vi "PWA_Setup_Panel.vi"(0 "Show Panel?":bool, 1 "Check Calib file?":bool, 2 "OK":T1, 3 "Incoming Setup String":string) -> (7 "Outgoing Setup String":string)   [LabVIEW 2022 SP3]
uses:
  Controls/ok_button.ctl
  File/Setup_Filetype.ctl
  Controls/Post_Process.ctl
  Controls/App_Global.ctl
  Controls/Inst_type.ctl
  Globals/Meas_global.vi
  PWAtasksGLOBAL.vi
panel:
  in  "Probe Rotated Thro' 180":bool
  in  "Software + buffering delay per pulse (s)":dbl=9.7e-06
  in  "Symbol":string
  in  "Pulse length \nx2 micro sec":i16=1 min=1 max=12
  in  "Clock Rate":bool
  in  "Gain":i16=1 min=1 max=12
  in  "Wire Current mA":i16(knob)=1 min=1 max=3 step=1 scale=1.0..3.0
  in  "Trigger -ve":dbl(knob)=1.0 min=0.0 max=5.0 scale=0.0..5.0 scale format="%#.2f"
  in  "Trigger +ve":dbl(knob)=1.0 min=0.0 max=5.0 scale=0.0..5.0 scale format="%#.2f"
  out "Calib Path from file":path
  in  "Use Latest":bool=TRUE
  in  "PWA Calib. File Path":path=path "/G5_1_HD/Users/paulhayden/Desktop/Labview test/PWA_Calib.xls"
  in  "Minimum TOF (mu.s)":i16=225
  in  "PWA Freq. (Hz)":dbl=30.0 min=0.0 max=50.0
  # "PELA Flow Instruments Ltd."
  # "TRIGGER LEVELS\n(volts)"
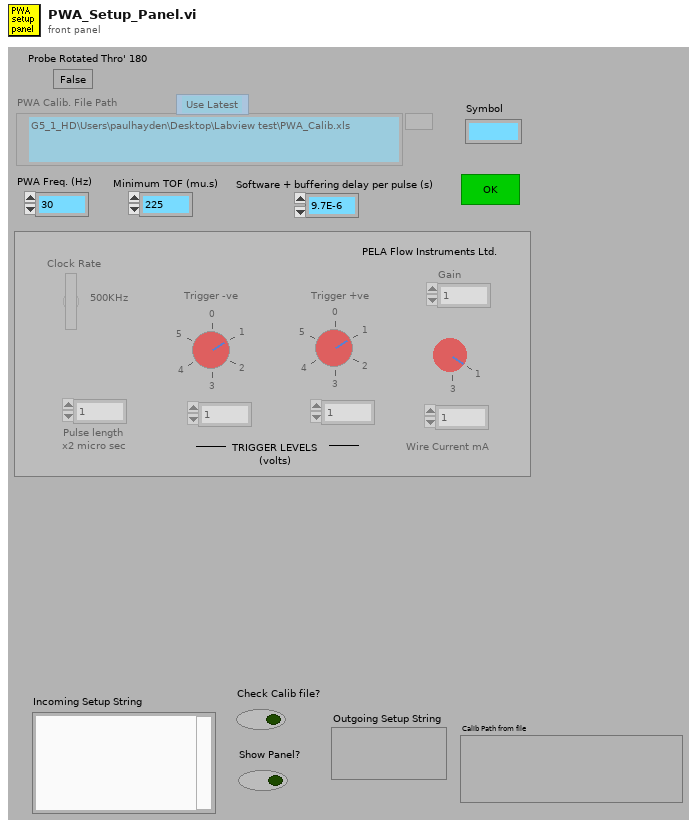
[diagram p1: front panel]
types:
  T1 = typedef "ok_button.ctl" = bool
  T2 = typedef "Setup_Filetype.ctl" = enum16{"Measurement Setups", "Calibration Setups", "General", "Results File Plotter Setups", "Speed Calib Tweaks"}
  T3 = typedef "Post_Process.ctl" = enum16{"Take New Data", "Post Process Raw Data File"}
  T4 = typedef "App_Global.ctl" = enum16{"Read Global", "Write to Global", "Initialise Array"}
  T5 = typedef "Inst_type.ctl" = enum16{"Raw voltage", "Raw with zero offsetting", "Propeller anemometer", "Pressure Transducer", "Pitot-static tube", "Hot wire", "Cross wire 1", "Cross wire 2", "Generic Linear", "Generic Polynomial", "Generic BackPoly", "Fast FID", "Thermocouple", "Cold wire", "Pulsed Wire", "LDA Vel", "LDA Tran time", "LDA Arr time", "Microphone"}
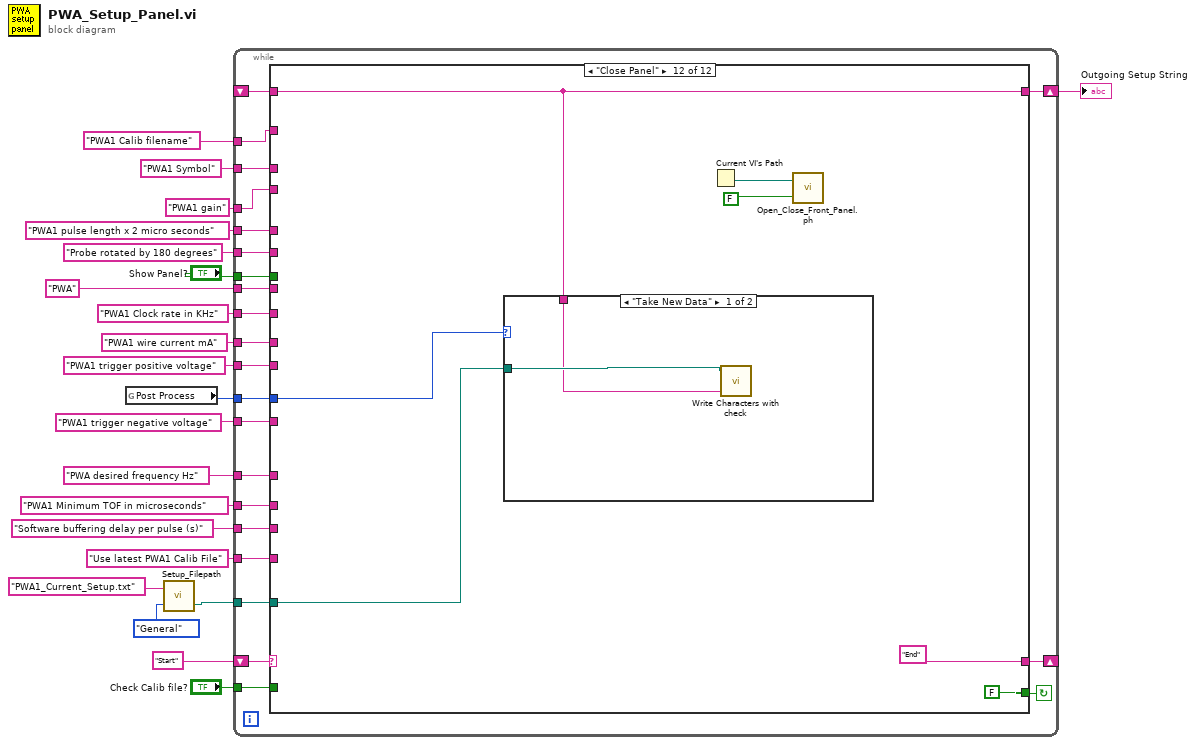
[diagram p0: block diagram]
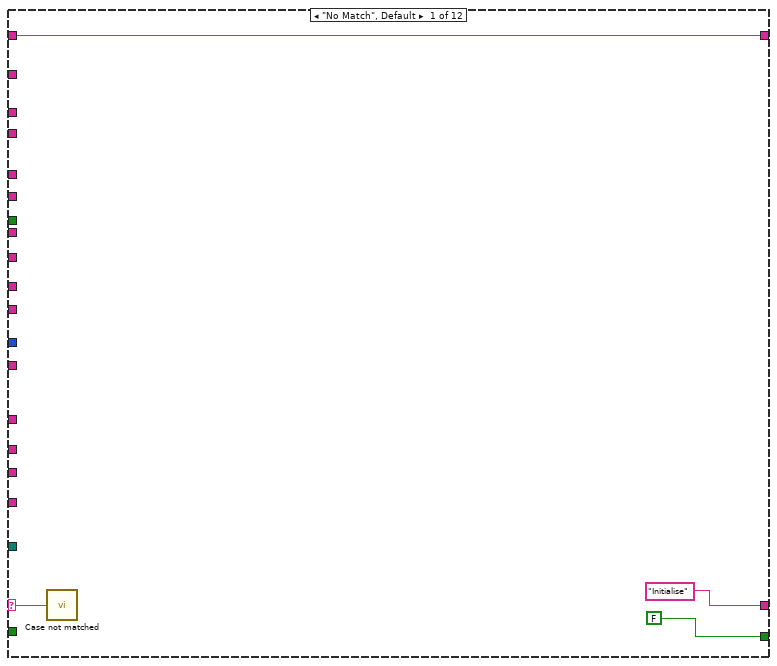
[diagram p2: hidden frame]
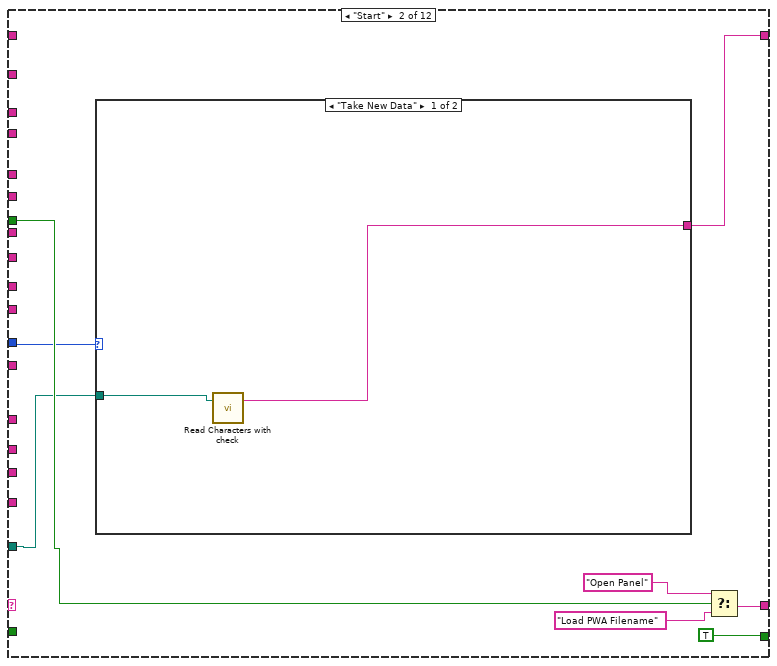
[diagram p3: hidden frame]
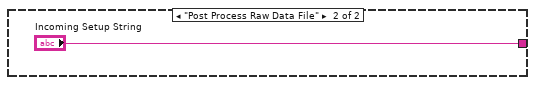
[diagram p4: hidden frame]
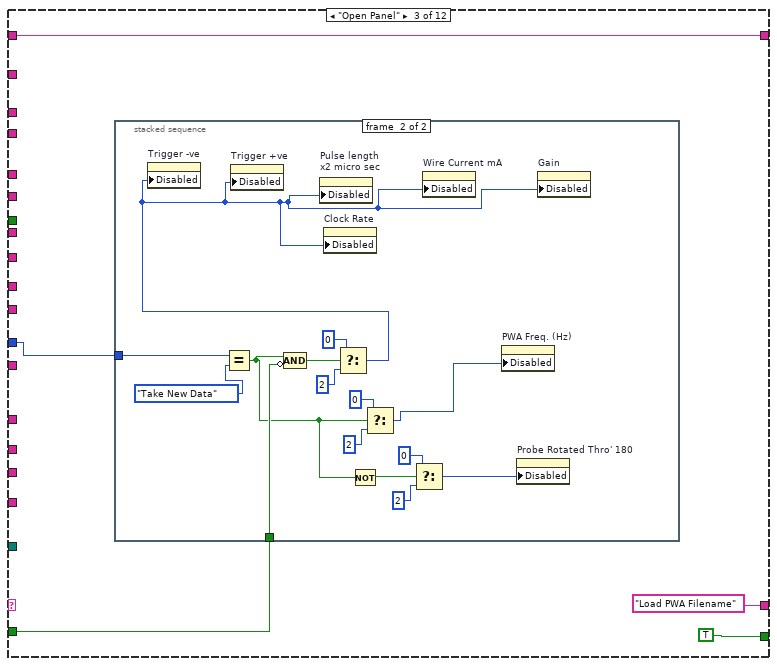
[diagram p5: hidden frame]
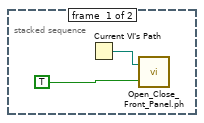
[diagram p6: hidden frame]
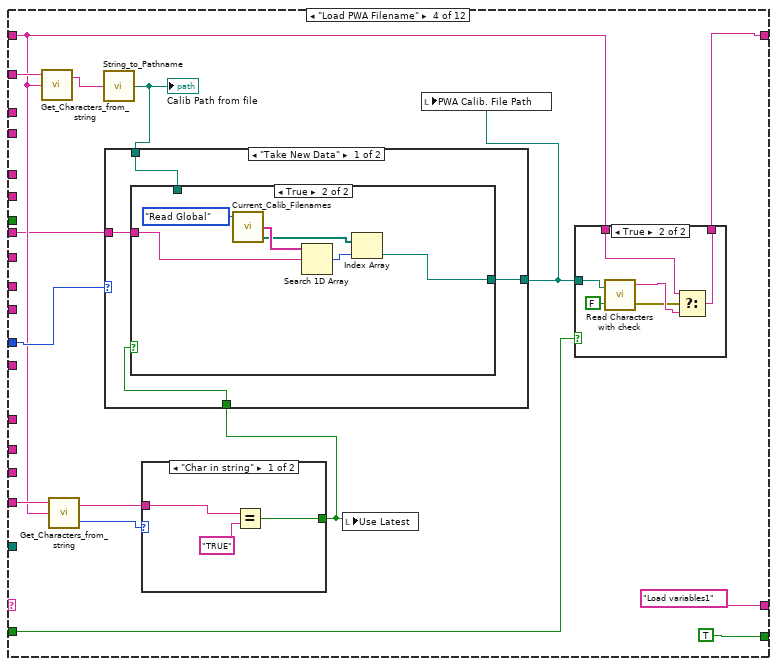
[diagram p7: hidden frame]
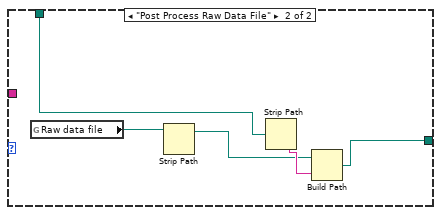
[diagram p10: hidden frame]
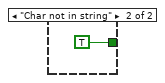
[diagram p11: hidden frame]
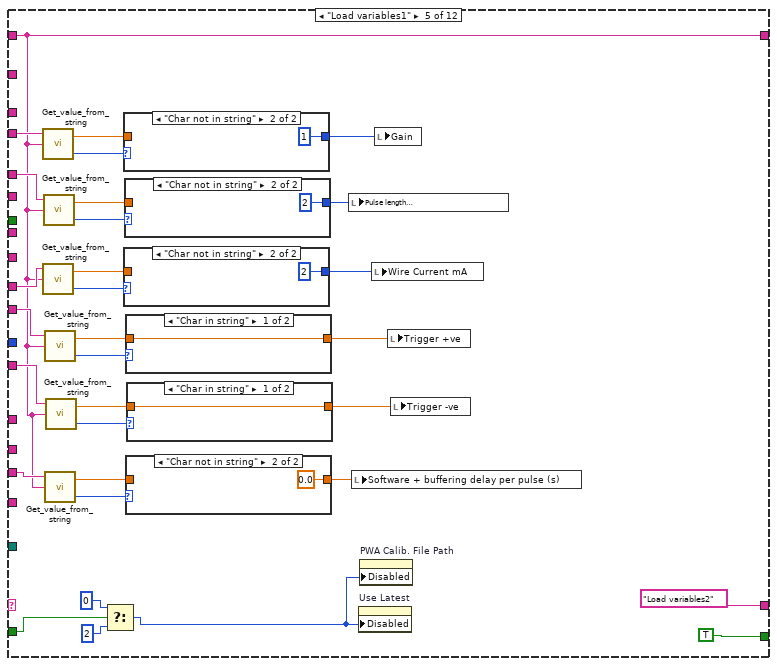
[diagram p12: hidden frame]
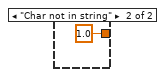
[diagram p14: hidden frame]
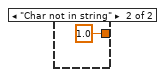
[diagram p15: hidden frame]
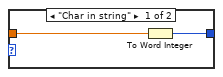
[diagram p16: hidden frame]
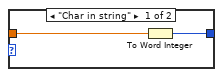
[diagram p17: hidden frame]
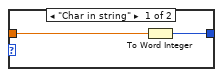
[diagram p18: hidden frame]
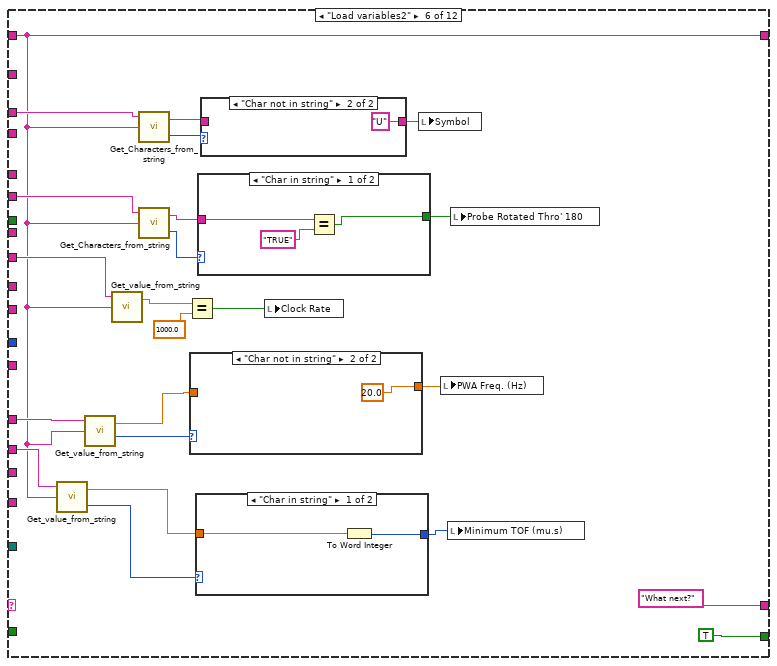
[diagram p19: hidden frame]
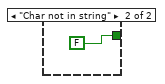
[diagram p20: hidden frame]
diagram:
  n1 = global read "Meas_global.vi" "Post Process"() -> (w20:T3)
  n2 = call "Setup_Filepath.vi"("Setup File Type"=Setup_Filetype."General", "Filename in"="PWA1_Current_Setup.txt" ("name or relative path")) -> ("Filename Out"=w2:path)  [unwired: 1 out]
  n3 = while {
    shift-left: "Start" -> [w43]
    shift-right: [w44] -> _
    tunnel: "Show Panel?" -> [w42]
    tunnel: w20 -> [w41]
    tunnel: "PWA1 Calib filename" -> [w39]
    tunnel: "Use latest PWA1 Calib File" -> [w40]
    tunnel: "PWA1 Minimum TOF in microseconds" -> [w38]
    tunnel: "PWA desired frequency Hz" -> [w37]
    tunnel: "Check Calib file?" -> [w36]
    tunnel: "PWA1 gain" -> [w35]
    tunnel: "PWA1 pulse length x 2 micro seconds" -> [w34]
    tunnel: "PWA1 wire current mA" -> [w33]
    tunnel: "PWA1 trigger positive voltage" -> [w32]
    tunnel: "PWA1 trigger negative voltage" -> [w31]
    tunnel: "PWA1 Clock rate in KHz" -> [w30]
    shift-right: [w29] -> w7
    shift-left: _ -> [w28]
    tunnel: "PWA1 Symbol" -> [w27]
    tunnel: w2 -> [w26]
    tunnel: "Software buffering delay per pulse (s)" -> [w25]
    tunnel: "Probe rotated by 180 degrees" -> [w24]
    tunnel: "PWA" ("element") -> [w23]
    stop <- w45 continue-if-true
    n4 = case shown="\"Close Panel\"" w43 {
      selector: w43 -> [w46 _ _ _ _ _ _ _ _ _ _ _]
      tunnel: [FALSE TRUE TRUE TRUE TRUE TRUE TRUE TRUE ("Show Panel?") TRUE ("Show Panel?") TRUE ("Show Panel?") w334 FALSE ("Show Panel?")] -> w45
      tunnel: ["Initialise" w50 "Load PWA Filename" "Load variables1" "Load variables2" "What next?" w212 "Save PWA values" "2nd Save PWA values" "PWA Setup Summary" "Close Panel" "End"] -> w44
      tunnel: w42 -> [_ w56 _ _ _ _ _ _ _ _ w334 _]
      tunnel: w41 -> [_ w53 w63 w89 _ _ w214 _ _ _ _ w336]
      tunnel: w40 -> [_ _ _ w91 _ _ _ _ w272 _ _ _]
      tunnel: w39 -> [_ _ _ w94 _ _ _ _ w282 _ _ _]
      tunnel: w38 -> [_ _ _ _ _ w191 _ _ w280 _ _ _]
      tunnel: w37 -> [_ _ _ _ _ w190 _ _ w281 _ _ _]
      tunnel: w36 -> [_ _ w61 w86 w153 _ w210 _ _ _ _ _]
      tunnel: w35 -> [_ _ _ _ w146 _ _ _ _ w319 _ _]
      tunnel: w34 -> [_ _ _ _ w142 _ _ _ _ w303 _ _]
      tunnel: w33 -> [_ _ _ _ w130 _ _ _ _ w308 _ _]
      tunnel: w32 -> [_ _ _ _ w135 _ _ _ _ w305 _ _]
      tunnel: w31 -> [_ _ _ _ w131 _ _ _ _ w304 _ _]
      tunnel: w30 -> [_ _ _ _ _ w183 _ _ _ w314 _ _]
      tunnel: [w47 w52 w62 w84 w126 w174 w209 w244 w268 w294 w324 w340] -> w29
      tunnel: w28 -> [w47 _ w62 w85 w126 w174 w209 w244 _ w295 w324 w340]
      tunnel: w27 -> [_ _ _ _ _ w179 _ _ w266 _ _ _]
      tunnel: w26 -> [_ w51 _ _ _ _ _ _ _ _ _ w339]
      tunnel: w25 -> [_ _ _ _ w127 _ _ _ _ w292 _ _]
      tunnel: w24 -> [_ _ _ _ _ w175 _ _ w259 _ _ _]
      tunnel: w23 -> [_ _ _ w83 _ _ w205 w239 _ _ _ _]
      frame "No Match", Default {
        n5 = call "Case not matched.vi"("Case Name not Matched"=w46) -> ()
      }
      frame "Start" {
        n6 = case shown="\"Take New Data\"" w53 {
          tunnel: [w58 "Incoming Setup String"] -> w52
          tunnel: w51 -> [w59 _]
          frame "Take New Data" {
            n7 = call "Read Characters with check.vi"("file (use dialog)"=w59) -> ("Read String"=w58:string)  [unwired: 1 in, 1 out]
          }
          frame "Post Process Raw Data File" {
          }
        }
        n8 = Select(t="Open Panel", s=w56, f="Load PWA Filename") -> (s? t:f=w50:string)
      }
      frame "Open Panel" {
        n9 = stacked-sequence {
          tunnel: w63 -> [_ w82]
          tunnel: w61 -> [_ w77]
          frame #0 {
            n10 = Current VI's Path() -> (path=w67:path)
            n11 = call "Open_Close_Front_Panel.ph.vi"("openWindow (T)"=TRUE ("Front Panel Window:Open"), "VI path"=w67) -> ()  [unwired: 1 in, 1 out]
          }
          frame #1 {
            n12 = Equal?(x=w82, y=Post_Process."Take New Data" ("Post Process")) -> (x = y?=w70:bool)
            n13 = Compound Arithmetic op=AND(w70, invert w77) -> (w76:bool)
            n14 = Select(t=u8 0 ("Disabled"), s=w76, f=u8 2) -> (s? t:f=w78:u8)
            n15 = property on="Trigger -ve" class="Knob (strict)"("Disabled"=w78) -> ()  [unwired: 2 in, 2 out]
            n16 = property on="Trigger +ve" class="Knob (strict)"("Disabled"=w78) -> ()  [unwired: 2 in, 2 out]
            n17 = property on="Pulse length \nx2 micro sec" class="DigNum (strict)"("Disabled"=w78) -> ()  [unwired: 2 in, 2 out]
            n18 = property on="Clock Rate" class="Bool (strict)"("Disabled"=w78) -> ()  [unwired: 2 in, 2 out]
            n19 = Not(x=w70) -> (.not. x?=w69:bool)
            n20 = Select(t=u8 0 ("Disabled"), s=w70, f=u8 2) -> (s? t:f=w73:u8)
            n21 = Select(t=u8 0 ("Disabled"), s=w69, f=u8 2) -> (s? t:f=w68:u8)
            n22 = property on="Wire Current mA" class="Knob (strict)"("Disabled"=w78) -> ()  [unwired: 2 in, 2 out]
            n23 = property on="PWA Freq. (Hz)" class="DigNum (strict)"("Disabled"=w73) -> ()  [unwired: 2 in, 2 out]
            n24 = property on="Probe Rotated Thro' 180" class="Bool (strict)"("Disabled"=w68) -> ()  [unwired: 2 in, 2 out]
            n25 = property on="Gain" class="DigNum (strict)"("Disabled"=w78) -> ()  [unwired: 2 in, 2 out]
          }
        }
      }
      frame "Load PWA Filename" {
        n26 = call "Get_Characters_from_string.vi"("Input string"=w85, "Variable name"=w94) -> ("Value"=w95:string)  [unwired: 1 in, 1 out]
        n27 = call "Get_Characters_from_string.vi"("Input string"=w85, "Variable name"=w91) -> ("Status"=w92:enum16{"Char in string", "Char not in string"}, "Value"=w93:string)  [unwired: 1 in]
        n28 = call "String_to_Pathname.vi"("Input String"=w95) -> ("path"=w90:path)
        "Calib Path from file" <- w90
        n29 = case shown="\"Char in string\"" w92 {
          tunnel: w93 -> [w123 _]
          tunnel: [w121 TRUE] -> w88
          frame "Char in string" {
            n30 = Equal?(x=w123, y="TRUE") -> (x = y?=w121:bool)
          }
          frame "Char not in string" {
          }
        }
        n31 = case shown="\"Take New Data\"" w89 {
          tunnel: [w107 w116] -> w87
          tunnel: w90 -> [w106 w119]
          tunnel: w88 -> [w108 _]
          tunnel: w83 -> [w105 _]
          frame "Take New Data" {
            n32 = case shown="True" w108 {
              tunnel: [w109 w111] -> w107
              tunnel: w106 -> [w109 _]
              tunnel: w105 -> [_ w110]
              frame False {
              }
              frame True {
                n33 = call "Current_Calib_Filenames.vi"("Mode"=App_Global."Read Global") -> ("Calib Filename Out"=w113:path[], "Channel ID Output"=w114:string[])  [unwired: 2 in, 1 out]
                n34 = Search 1D Array(1D array=w114, element=w110) -> (index of element=w112:i32)  [unwired: 1 out]
                n35 = Index Array(array=w113, index=w112) -> (element=w111:path)
              }
            }
          }
          frame "Post Process Raw Data File" {
            n36 = global read "Meas_global.vi" "Raw data file"() -> (w120:path)
            n37 = Strip Path(path=w120) -> (stripped path=w117:path)  [unwired: 1 out]
            n38 = Strip Path(path=w119) -> (name=w118:string)  [unwired: 1 out]
            n39 = Build Path(base path=w117, name or relative path=w118) -> (appended path=w116:path)
          }
        }
        n40 = local write "Use Latest"(w88) -> ()
        n41 = local write "PWA Calib. File Path"(w87) -> ()
        n42 = case shown="True" w86 {
          tunnel: w87 -> [_ w100]
          tunnel: w85 -> [w98 w104]
          tunnel: [w98 w103] -> w84
          frame False {
          }
          frame True {
            n43 = call "Read Characters with check.vi"("Call EnFlo Error Handler?"=FALSE, "file (use dialog)"=w100) -> ("error out"=w101:errorcluster, "Read String"=w102:string)
            n44 = Select(t=w104, s=w101, f=w102) -> (s? t:f=w103:string)
          }
        }
      }
      frame "Load variables1" {
        n45 = call "Get_value_from_string.vi"("Input string"=w126, "Variable name"=w146) -> ("Status"=w148:enum16{"Char in string", "Char not in string"}, "Value"=w149:dbl)  [unwired: 1 in]
        n46 = call "Get_value_from_string.vi"("Input string"=w126, "Variable name"=w130) -> ("Status"=w140:enum16{"Char in string", "Char not in string"}, "Value"=w141:dbl)  [unwired: 1 in]
        n47 = call "Get_value_from_string.vi"("Input string"=w126, "Variable name"=w142) -> ("Status"=w144:enum16{"Char in string", "Char not in string"}, "Value"=w143:dbl)  [unwired: 1 in]
        n48 = call "Get_value_from_string.vi"("Input string"=w126, "Variable name"=w135) -> ("Status"=w137:enum16{"Char in string", "Char not in string"}, "Value"=w136:dbl)  [unwired: 1 in]
        n49 = call "Get_value_from_string.vi"("Input string"=w126, "Variable name"=w127) -> ("Status"=w128:enum16{"Char in string", "Char not in string"}, "Value"=w125:dbl)  [unwired: 1 in]
        n50 = call "Get_value_from_string.vi"("Input string"=w126, "Variable name"=w131) -> ("Status"=w133:enum16{"Char in string", "Char not in string"}, "Value"=w134:dbl)  [unwired: 1 in]
        n51 = Select(t=u8 0 ("Disabled"), s=w153, f=u8 2 ("Disabled")) -> (s? t:f=w150:u8)
        n52 = case shown="\"Char not in string\"" w148 {
          tunnel: w149 -> [w169 _]
          tunnel: [w168 i16 1 ("PWA No. of Samples")] -> w147
          frame "Char in string" {
            n53 = To Word Integer(number=w169) -> (16bit integer=w168:i16)
          }
          frame "Char not in string" {
          }
        }
        n54 = case shown="\"Char not in string\"" w140 {
          tunnel: w141 -> [w163 _]
          tunnel: [w162 i16 2 ("PWA No. of Samples")] -> w139
          frame "Char in string" {
            n55 = To Word Integer(number=w163) -> (16bit integer=w162:i16)
          }
          frame "Char not in string" {
          }
        }
        n56 = case shown="\"Char not in string\"" w144 {
          tunnel: w143 -> [w166 _]
          tunnel: [w165 i16 2 ("PWA No. of Samples")] -> w145
          frame "Char in string" {
            n57 = To Word Integer(number=w166) -> (16bit integer=w165:i16)
          }
          frame "Char not in string" {
          }
        }
        n58 = case shown="\"Char in string\"" w137 {
          tunnel: w136 -> [w160 _]
          tunnel: [w160 1.0 ("Value")] -> w138
          frame "Char in string" {
          }
          frame "Char not in string" {
          }
        }
        n59 = case shown="\"Char not in string\"" w128 {
          tunnel: w125 -> [w156 _]
          tunnel: [w156 0.0 ("Value")] -> w129
          frame "Char in string" {
          }
          frame "Char not in string" {
          }
        }
        n60 = case shown="\"Char in string\"" w133 {
          tunnel: w134 -> [w158 _]
          tunnel: [w158 1.0 ("Value")] -> w132
          frame "Char in string" {
          }
          frame "Char not in string" {
          }
        }
        n61 = local write "Pulse length \nx2 micro sec"(w145) -> ()
        n62 = local write "Software + buffering delay per pulse (s)"(w129) -> ()
        n63 = property on="Use Latest" class="Bool (strict)"("Disabled"=w150) -> ()  [unwired: 2 in, 2 out]
        n64 = property on="PWA Calib. File Path" class="Path"("Disabled"=w150) -> ()  [unwired: 2 in, 2 out]
        n65 = local write "Wire Current mA"(w139) -> ()
        n66 = local write "Gain"(w147) -> ()
        n67 = local write "Trigger +ve"(w138) -> ()
        n68 = local write "Trigger -ve"(w132) -> ()
      }
      frame "Load variables2" {
        n69 = call "Get_value_from_string.vi"("Input string"=w174, "Variable name"=w191) -> ("Status"=w186:enum16{"Char in string", "Char not in string"}, "Value"=w185:dbl)  [unwired: 1 in]
        n70 = call "Get_value_from_string.vi"("Input string"=w174, "Variable name"=w190) -> ("Status"=w189:enum16{"Char in string", "Char not in string"}, "Value"=w188:dbl)  [unwired: 1 in]
        n71 = call "Get_value_from_string.vi"("Input string"=w174, "Variable name"=w183) -> ("Value"=w182:dbl)  [unwired: 1 in, 1 out]
        n72 = call "Get_Characters_from_string.vi"("Input string"=w174, "Variable name"=w179) -> ("Status"=w178:enum16{"Char in string", "Char not in string"}, "Value"=w177:string)  [unwired: 1 in]
        n73 = call "Get_Characters_from_string.vi"("Input string"=w174, "Variable name"=w175) -> ("Status"=w173:enum16{"Char in string", "Char not in string"}, "Value"=w171:string)  [unwired: 1 in]
        n74 = Equal?(x=w182, y=1000.0) -> (x = y?=w180:bool)
        n75 = case shown="\"Char not in string\"" w189 {
          tunnel: w188 -> [w203 _]
          tunnel: [w203 20.0 ("PWA No. of Samples")] -> w187
          frame "Char in string" {
          }
          frame "Char not in string" {
          }
        }
        n76 = case shown="\"Char in string\"" w186 {
          tunnel: w185 -> [w201 _]
          tunnel: [w200 i16 225 ("Minimum TOF (mu.s)")] -> w184
          frame "Char in string" {
            n77 = To Word Integer(number=w201) -> (16bit integer=w200:i16)
          }
          frame "Char not in string" {
          }
        }
        n78 = case shown="\"Char in string\"" w173 {
          tunnel: [w194 FALSE] -> w172
          tunnel: w171 -> [w196 _]
          frame "Char in string" {
            n79 = Equal?(x=w196, y="TRUE") -> (x = y?=w194:bool)
          }
          frame "Char not in string" {
          }
        }
        n80 = case shown="\"Char not in string\"" w178 {
          tunnel: w177 -> [w198 _]
          tunnel: [w198 "U" ("Value")] -> w176
          frame "Char in string" {
          }
          frame "Char not in string" {
          }
        }
        n81 = local write "Clock Rate"(w180) -> ()
        n82 = local write "Symbol"(w176) -> ()
        n83 = local write "PWA Freq. (Hz)"(w187) -> ()
        n84 = local write "Minimum TOF (mu.s)"(w184) -> ()
        n85 = local write "Probe Rotated Thro' 180"(w172) -> ()
      }
      frame "What next?" {
        n86 = local read "PWA Calib. File Path"() -> (w208:path)
        n87 = case shown="\"Take New Data\"" w214 {
          tunnel: [w225 w234] -> w206
          tunnel: w208 -> [w224 w237]
          tunnel: "Use Latest" -> [w226 _]
          tunnel: w205 -> [w223 _]
          frame "Take New Data" {
            n88 = case shown="True" w226 {
              tunnel: [w227 w229] -> w225
              tunnel: w224 -> [w227 _]
              tunnel: w223 -> [_ w228]
              frame False {
              }
              frame True {
                n89 = call "Current_Calib_Filenames.vi"("Mode"=App_Global."Read Global") -> ("Calib Filename Out"=w231:path[], "Channel ID Output"=w232:string[])  [unwired: 2 in, 1 out]
                n90 = Search 1D Array(1D array=w232, element=w228) -> (index of element=w230:i32)  [unwired: 1 out]
                n91 = Index Array(array=w231, index=w230) -> (element=w229:path)
              }
            }
          }
          frame "Post Process Raw Data File" {
            n92 = global read "Meas_global.vi" "Raw data file"() -> (w238:path)
            n93 = Strip Path(path=w238) -> (stripped path=w235:path)  [unwired: 1 out]
            n94 = Strip Path(path=w237) -> (name=w236:string)  [unwired: 1 out]
            n95 = Build Path(base path=w235, name or relative path=w236) -> (appended path=w234:path)
          }
        }
        n96 = case shown="True" "OK" {
          tunnel: ["What next?" ("f") w220] -> w212
          tunnel: w210 -> [_ w219]
          frame False {
            n97 = Wait (ms)(milliseconds to wait=u32 300) -> ()  [unwired: 1 out]
          }
          frame True {
            n98 = Select(t="Check Calib File", s=w219, f="Save PWA values") -> (s? t:f=w220:string)
          }
        }
        n99 = Not Equal?(x=w208, y=w206) -> (x != y?=w207:bool)
        n100 = case shown="False" w207 {
          tunnel: w206 -> [_ w216]
          frame False {
          }
          frame True {
            n101 = local write "PWA Calib. File Path"(w216) -> ()
          }
        }
      }
      frame "Check Calib File" {
        n102 = local read "Use Latest"() -> (w240:bool)
        n103 = local read "PWA Calib. File Path"() -> (w243:path)
        n104 = call "Find_calibration_file.vi"("Inst type"=Inst_type."Pulsed Wire", "Channel ID"=w239, "Use Latest Calib"=w240, "filename"=w243) -> ("filename out"=w242:path)
        n105 = Not Equal?(x=w242, y=w243) -> (x != y?=w246:bool)
        n106 = And(x=w246, y=w240) -> (x .and. y?=w245:bool)
        n107 = local write "PWA Calib. File Path"(w242) -> ()
        n108 = case shown="True" w245 {
          tunnel: w242 -> [_ w250]
          tunnel: w239 -> [_ w249]
          frame False {
          }
          frame True {
            n109 = Build Array(w250) -> (w253:path[])
            n110 = Build Array(w249) -> (w252:string[])
            n111 = call "Current_Calib_Filenames.vi"("Calib Filename"=w253, "Channel ID input"=w252, "Mode"=App_Global."Write to Global") -> ()  [unwired: 3 out]
          }
        }
      }
      frame "Save PWA values" {
        n112 = local read "Use Latest"() -> (w276:bool)
        n113 = global write "PWAtasksGLOBAL.vi" "PWA Freq. (Hz)"("PWA Freq. (Hz)") -> ()
        n114 = global write "PWAtasksGLOBAL.vi" "PWA Calib. File Path"("PWA Calib. File Path") -> ()
        n115 = Select(t="TRUE", s=w276, f="FALSE") -> (s? t:f=w273:string)
        n116 = global write "PWAtasksGLOBAL.vi" "PWA Symbol"("Symbol") -> ()
        n117 = call "Characters_to_string.vi"("Characters to write"="Symbol", "Label for characters"=w266) -> ("Output string"=w265:string)  [unwired: 1 in]
        n118 = call "Characters_to_string.vi"("Characters to write"=w273, "Label for characters"=w272) -> ("Output string"=w271:string)  [unwired: 1 in]
        n119 = call "Value_to_string.vi"("Value"="PWA Freq. (Hz)", "Label for value"=w281) -> ("Output string"=w278:string)  [unwired: 1 in]
        n120 = global write "PWAtasksGLOBAL.vi" "Probe Rotated Thro' 180"("Probe Rotated Thro' 180") -> ()
        n121 = call "Path_2_String.vi"("Real Path"="PWA Calib. File Path") -> ("Path String"=w283:string)
        n122 = Select(t="TRUE" ("y"), s="Probe Rotated Thro' 180", f="FALSE") -> (s? t:f=w255:string)
        n123 = call "Characters_to_string.vi"("Characters to write"=w255, "Label for characters"=w259) -> ("Output string"=w256:string)  [unwired: 1 in]
        n124 = call "Characters_to_string.vi"("Characters to write"=w283, "Label for characters"=w282) -> ("Output string"=w279:string)  [unwired: 1 in]
        n125 = local read "Clock Rate"() -> (w263:bool)
        n126 = case shown="True" w263 {
          tunnel: [w286 w290] -> w262
          tunnel: [w285 w290] -> w261
          tunnel: "Minimum TOF (mu.s)" -> [w288 w290]
          frame False {
            w287 = i16 2 ("y")
            n127 = Divide(x=w288, y=w287) -> (x/y=w289:dbl)
            n128 = To Word Integer(number=w289) -> (16bit integer=w286:i16)
            n129 = Multiply(x=w286, y=w287) -> (x*y=w285:i16)
          }
          frame True {
          }
        }
        n130 = call "Value_to_string.vi"("Value"=w261, "Label for value"=w280) -> ("Output string"=w277:string)  [unwired: 1 in]
        n131 = Concatenate Strings(w279, w265, w256, w278, w277, w271) -> (w268:string)
        n132 = global write "PWAtasksGLOBAL.vi" "Minimum TOF Index"(w262) -> ()
      }
      frame "2nd Save PWA values" {
        n133 = Select(t=1000.0, s="Clock Rate", f=500.0) -> (s? t:f=w313:dbl)
        n134 = call "Value_to_string.vi"("Value"="Gain", "Label for value"=w319) -> ("Output string"=w301:string)  [unwired: 1 in]
        n135 = call "Value_to_string.vi"("Value"="Trigger -ve", "Label for value"=w304) -> ("Output string"=w296:string)  [unwired: 1 in]
        n136 = call "Value_to_string.vi"("Value"="Wire Current mA", "Label for value"=w308) -> ("Output string"=w298:string)  [unwired: 1 in]
        n137 = call "Value_to_string.vi"("Value"="Trigger +ve", "Label for value"=w305) -> ("Output string"=w297:string)  [unwired: 1 in]
        n138 = call "Value_to_string.vi"("Value"="Pulse length \nx2 micro sec", "Label for value"=w303) -> ("Output string"=w300:string)  [unwired: 1 in]
        n139 = call "Value_to_string.vi"("Value"=w313, "Label for value"=w314) -> ("Output string"=w299:string)  [unwired: 1 in]
        n140 = Multiply(x=w313, y=1000.0) -> (x*y=w311:dbl)
        n141 = Reciprocal(x=w311) -> (1/x=w310:dbl)
        n142 = call "Value_to_string.vi"("Value"="Software + buffering delay per pulse (s)", "Label for value"=w292) -> ("Output string"=w291:string)  [unwired: 1 in]
        n143 = global write "PWAtasksGLOBAL.vi" "PWA Seconds per clock pulse"(w310) -> ()
        n144 = Concatenate Strings(w295, w301, w300, w299, w298, w297, w296, w291) -> (w294:string)
      }
      frame "PWA Setup Summary" {
        n145 = local read "Pulse length \nx2 micro sec"() -> (w329:i16)
        n146 = local read "Wire Current mA"() -> (w328:i16)
        n147 = local read "Clock Rate"() -> (w333:bool)
        n148 = local read "Trigger -ve"() -> (w331:dbl)
        n149 = local read "Trigger +ve"() -> (w330:dbl)
        n150 = local read "Gain"() -> (w327:i16)
        n151 = Select(t="1MHz", s=w333, f="500KHz") -> (s? t:f=w332:string)
        n152 = Format Into String(format string="Clock=%s; Trig -ve=%.2f; Trig +ve=%.2f; Pulse length=%dx2micro sec; wire current=%dmA; Gain=%d", w332, w331, w330, w329, w328, w327) -> (resulting string=w325:string)  [unwired: 2 in, 1 out]
        n153 = global write "PWAtasksGLOBAL.vi" "PWA Setup summary"(w325) -> ()
      }
      frame "Close Panel" {
        n154 = case shown="\"Take New Data\"" w336 {
          tunnel: w340 -> [w343 _]
          tunnel: w339 -> [w344 _]
          frame "Take New Data" {
            n155 = call "Write Characters with check.vi"("String to Write"=w343, "file (use dialog)"=w344) -> ()  [unwired: 2 in, 1 out]
          }
          frame "Post Process Raw Data File" {
          }
        }
        n156 = Current VI's Path() -> (path=w338:path)
        n157 = call "Open_Close_Front_Panel.ph.vi"("openWindow (T)"=FALSE ("Front Panel Window:Open"), "VI path"=w338) -> ()  [unwired: 1 in, 1 out]
      }
    }
  }
  "Outgoing Setup String" <- w7
